vi "WiFi.vi"(0 "New WIFI Name":string="Honor V10", 1 "DelayTime (s)":dbl=1.0 caption="ConfigTime", 3 "配置连接次数":i32=5, 5 "Delay":string="2", 7 "超时时间":u32=25000, 9 "password":string="88888888", 11 "error in":errorcluster caption="error in (no error)", 13 "ping次数":string="6", 14 "ModelNumber":string) -> (4 "Acess":bool, 10 "TotalOut":string, 15 "error out":errorcluster caption="错误输出")   [LabVIEW 2013]
uses:
  <vilib>/Utility/sysdir.llb/System Directory Type.ctl
panel:
  out "数值":i32
  out "Time":u32
  out "新文本":string
  out "原文本":string
  out "STDping":string="WIFI名："
  out "standard output  2":string caption="标准输出"
  out "standard output  3":string caption="标准输出"
  out "SD":path caption="系统目录"
  out "standard output":string caption="标准输出"
  # "第一步，断开相应WIFI的连接\n第二步，替换配置文件\n第三步，添加配置文件到系统\n第四步，连接对应WIFI\n第五步，ping百度网址\n第六步，断开WIFI网络连接"
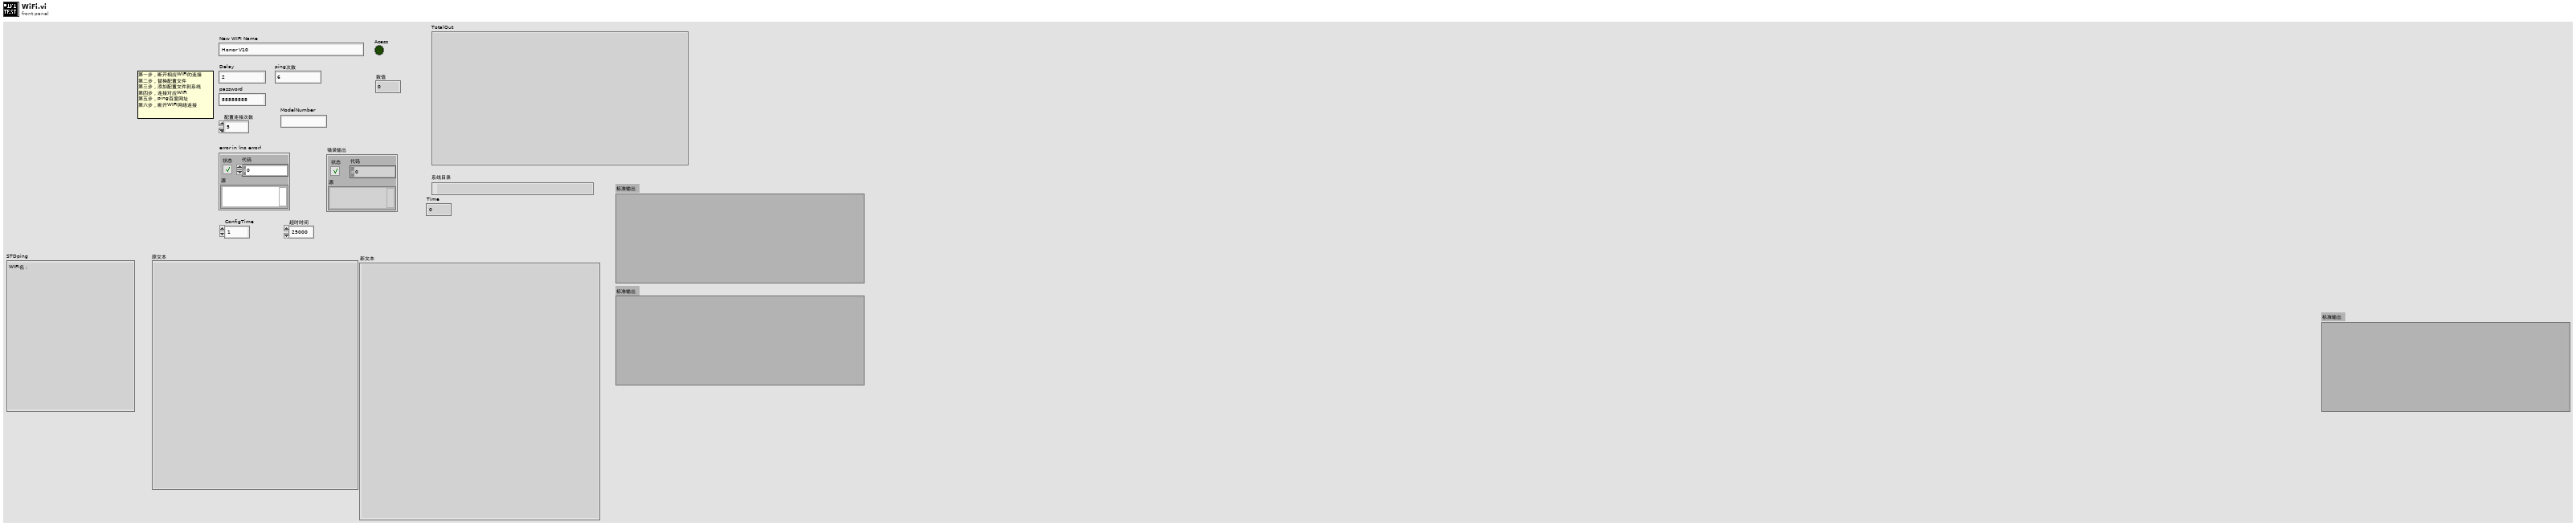
[diagram p1: front panel]
types:
  T1 = typedef "System Directory Type.ctl" = i32
  T2 = enum16{"open", "replace", "create", "open or create", "replace or create", "replace or create with confirmation"}
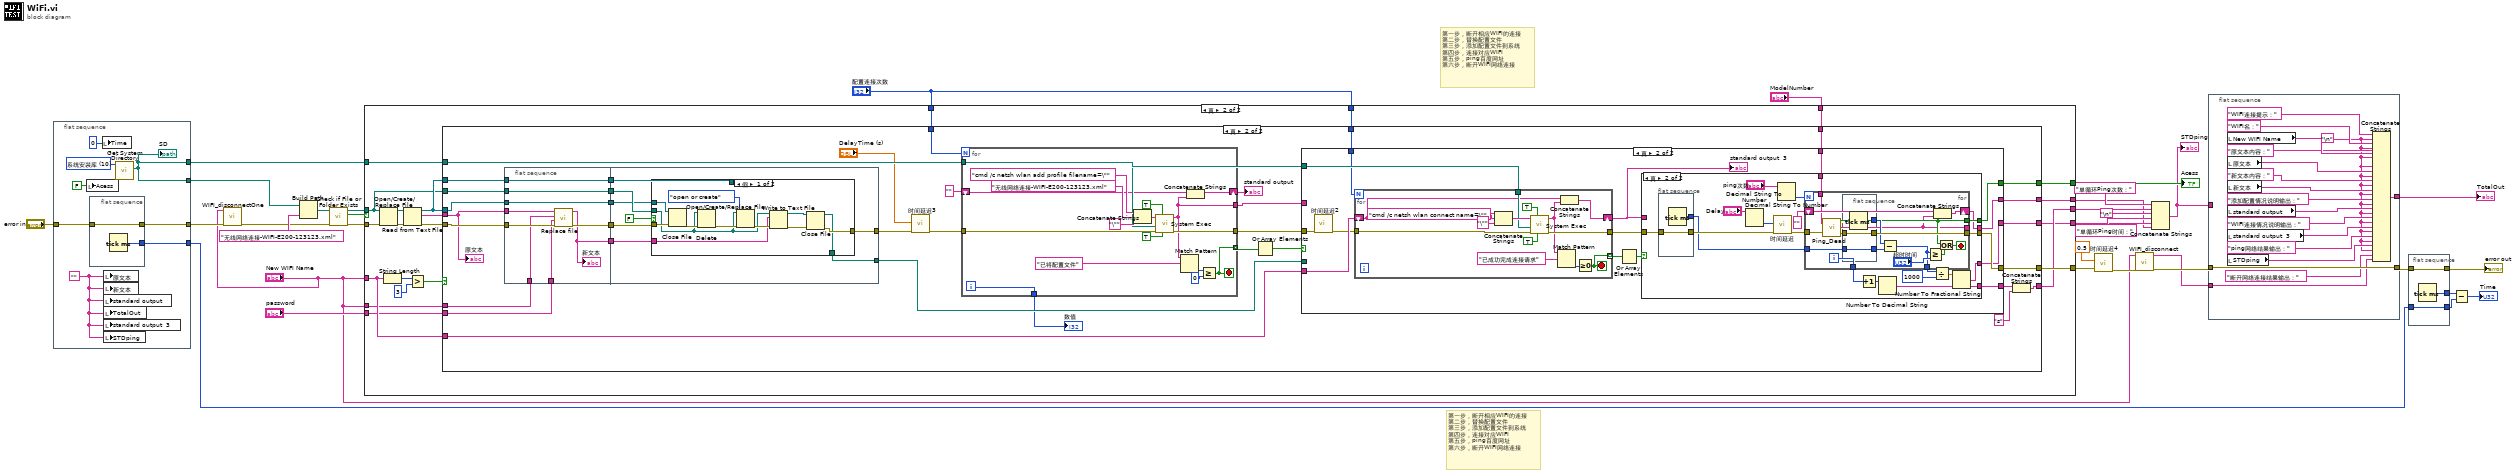
[diagram p0: block diagram]
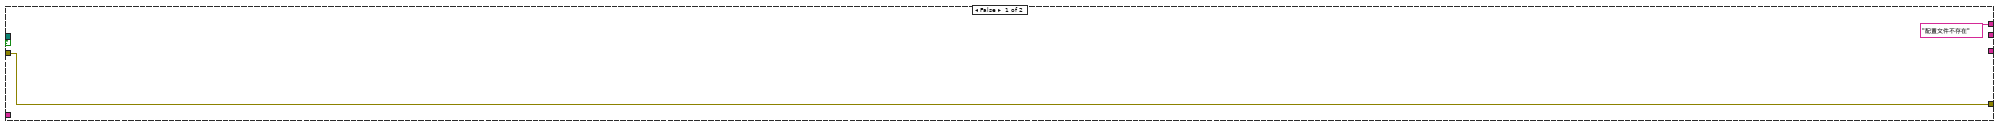
[diagram p2: hidden frame]
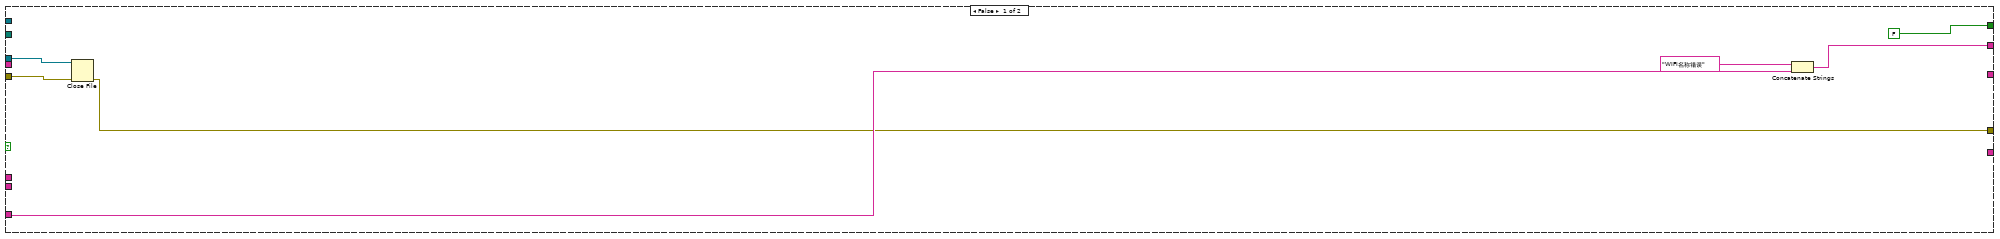
[diagram p3: hidden frame]
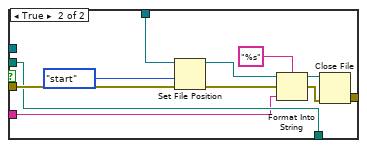
[diagram p4: hidden frame]
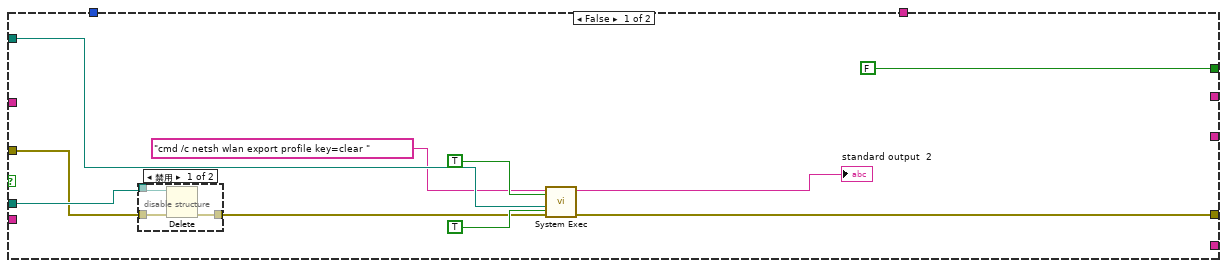
[diagram p5: hidden frame]
diagram:
  # "第一步，断开相应WIFI的连接\n第二步，替换配置文件\n第三步，添加配置文件到系统\n第四步，连接对应WIFI\n第五步，ping百度网址\n第六步，断开WIFI网络连接"
  # "第一步，断开相应WIFI的连接\n第二步，替换配置文件\n第三步，添加配置文件到系统\n第四步，连接对应WIFI\n第五步，ping百度网址\n第六步，断开WIFI网络连接"
  n1 = flat-sequence {
    tunnel: [w41] -> w31
    tunnel: [w41] -> w29
    tunnel: "error in" -> [w38]
    tunnel: [w39] -> w7
    tunnel: [w37] -> w16
    frame #0 {
      w40 = ""
      w42 = T1 10 items=["用户目录"=0, "用户桌面"=1, "用户文档"=2, "用户应用程序数据"=3, "用户设置"=4, "用户临时目录"=5, "公共文档"=6, "公共应用程序数据"=7, "公共设置"=8, "公共缓存"=13, "系统核心库"=9, "系统安装库"=10, "应用程序文件"=11, "启动盘根目录"=12] ("system directory type")
      n2 = local write "Acess"(FALSE ("Acess")) -> ()
      n3 = flat-sequence {
        tunnel: [w44] -> w39
        tunnel: w38 -> [w44]
        tunnel: [w43] -> w37
        frame #0 {
          n4 = Tick Count (ms)() -> (millisecond timer value=w43:u32)
        }
      }
      n5 = local write "Time"(u32 0 ("Time")) -> ()
      n6 = local write "原文本"(w40) -> ()
      n7 = local write "新文本"(w40) -> ()
      n8 = local write "standard output"(w40) -> ()
      n9 = local write "TotalOut"(w40) -> ()
      n10 = local write "standard output  3"(w40) -> ()
      n11 = local write "STDping"(w40) -> ()
      n12 = call <vilib>:"Get System Directory.vi"("system directory type"=w42) -> ("system directory"=w41:path)  [unwired: 10 in]
      "SD" <- w41
    }
  }
  n13 = call "WIFI_disconnectOne.vi"("错误输入"=w7, "WIFI_Name"="New WIFI Name") -> ("error out"=w8:errorcluster)  [unwired: 8 in, 1 out]
  n14 = Build Path(base path=w31, name or relative path="无线网络连接-WIFI-E200-123123.xml" ("名称或相对路径")) -> (appended path=w34:path)
  n15 = call <vilib>:"Check if File or Folder Exists.vi"("error in (no error)"=w8, "path"=w34) -> ("error out"=w32:errorcluster, "file or folder exists?"=w26:bool, "dup path"=w27:path)  [unwired: 7 in]
  n16 = case shown="真" w26 {
    tunnel: w32 -> [w45 w65]
    tunnel: w29 -> [_ w63]
    tunnel: "New WIFI Name" -> [_ w62]
    tunnel: [_ w60] -> w28
    tunnel: ["配置文件不存在" ("standard output") w59] -> w2
    tunnel: [w45 w55] -> w24
    tunnel: w27 -> [_ w54]
    tunnel: "password" -> [_ w53]
    tunnel: "New WIFI Name" -> [_ w52]
    tunnel: "配置连接次数" -> [_ w51]
    tunnel: "配置连接次数" -> [_ w50]
    tunnel: [_ w49] -> w11
    tunnel: [_ w48] -> w3
    tunnel: "ModelNumber" -> [_ w47]
    frame False {
    }
    frame True {
      n17 = Open/Create/Replace File(file path (use dialog)=w54, error in=w65) -> (refnum out=w68:refnum<file>, error out=w67:errorcluster)  [unwired: 4 in, 1 out]
      n18 = String Length(string=w62) -> (length=w58:i32)
      n19 = Read from Text File(file (use dialog)=w68, error in=w67) -> (refnum out=w61:refnum<file>, text=w64:string, error out=w66:errorcluster)  [unwired: 2 in, 1 out]
      n20 = Greater?(x=w58, y=3) -> (0:w56:bool)
      n21 = case shown="真" w56 {
        tunnel: w66 -> [w74 w94]
        tunnel: w61 -> [_ w109]
        tunnel: w64 -> [_ w89]
        tunnel: w62 -> [w73 w107]
        tunnel: w63 -> [_ w106]
        tunnel: w61 -> [w75 w101]
        tunnel: [w69 w105] -> w55
        tunnel: [FALSE ("Acess") w104] -> w60
        tunnel: [w71 w103] -> w59
        tunnel: w54 -> [_ w102]
        tunnel: w53 -> [_ w91]
        tunnel: w52 -> [_ w90]
        tunnel: w51 -> [_ w83]
        tunnel: w50 -> [_ w82]
        tunnel: [_ w78] -> w49
        tunnel: [_ w79] -> w48
        tunnel: w47 -> [_ w76]
        frame False {
          n22 = Close File(refnum=w75, error in=w74) -> (error out=w69:errorcluster)  [unwired: 1 out]
          n23 = Concatenate Strings("WIFI名称错误" ("字符串"), w73) -> (w71:string)
        }
        frame True {
          n24 = flat-sequence {
            tunnel: w101 -> [w134]
            tunnel: w102 -> [w135]
            tunnel: w109 -> [w136]
            tunnel: [w136] -> w97
            tunnel: [w135] -> w96
            tunnel: [w134] -> w95
            tunnel: w94 -> [w133]
            tunnel: [w132] -> w93
            tunnel: [w131] -> w92
            tunnel: w91 -> [w130]
            tunnel: w90 -> [w129]
            tunnel: w89 -> [w128]
            tunnel: [w144] -> w110
            tunnel: [w139] -> w98
            tunnel: w97 -> [w143]
            tunnel: w96 -> [w141]
            tunnel: w95 -> [w140]
            tunnel: w93 -> [w138]
            tunnel: w92 -> [w137]
            frame #0 {
              n25 = call "Replace file.vi"("error in"=w133, "password"=w130, "new wifi name"=w129, "txt input"=w128) -> ("error out"=w132:errorcluster, "txt output"=w131:string)  [unwired: 6 in]
              "新文本" <- w131
            }
            frame #1 {
              n26 = case shown="假" FALSE {
                tunnel: [w148 w162] -> w144
                tunnel: w138 -> [w155 w161]
                tunnel: w143 -> [_ w160]
                tunnel: w141 -> [w147 w158]
                tunnel: w140 -> [w156 _]
                tunnel: [w146 w158] -> w139
                tunnel: w137 -> [w145 w157]
                frame False {
                  n27 = Close File(refnum=w156, error in=w155) -> (error out=w154:errorcluster)  [unwired: 1 out]
                  n28 = Delete(path (use dialog)=w147, error in=w154) -> (error out=w152:errorcluster)  [unwired: 3 in, 2 out]
                  n29 = Open/Create/Replace File(file path (use dialog)=w147, error in=w152, operation (0:open)=T2."open or create" ("操作(0:open)")) -> (error out=w151:errorcluster)  [unwired: 3 in, 2 out]
                  n30 = Write to Text File(file (use dialog)=w147, text=w145, error in=w151) -> (refnum out=w150:refnum<file>, error out=w149:errorcluster)  [unwired: 1 in, 1 out]
                  n31 = Close File(refnum=w150, error in=w149) -> (path=w146:path, error out=w148:errorcluster)
                }
                frame True {
                  n32 = Set File Position(refnum=w160, from (0:start)=enum16{"start", "end", "current"}."start" ("自（0:起始）"), error in=w161) -> (refnum out=w163:refnum<file>, error out=w166:errorcluster)  [unwired: 1 in]
                  n33 = Format Into String(format string="%s" ("格式字符串"), initial string=w163, error in=w166, w157) -> (resulting string=w159:refnum<file>, error out=w165:errorcluster)
                  n34 = Close File(refnum=w159, error in=w165) -> (error out=w162:errorcluster)  [unwired: 1 out]
                }
              }
            }
          }
          n35 = call "时间延迟3"("error in (no error)"=w110, "Delay Time (s)"="DelayTime (s)") -> ("error out"=w100:errorcluster)  [unwired: 9 in]
          n36 = for {
            N: w83 -> [_]
            tunnel: [w121] -> w108
            tunnel: w106 -> [w120]
            tunnel: w100 -> [w119]
            shift-right: [w117] -> w87
            shift-left: "" -> [w118]
            tunnel: [w116] -> w84
            tunnel: [w112] -> w86 mode=indexing
            tunnel: [w111] -> w81
            i -> [w111]
            stop <- w112 stop-if-true
            n37 = Concatenate Strings("cmd /c netsh wlan add profile filename=\"" ("command line"), "无线网络连接-WIFI-E200-123123.xml" ("名称或相对路径"), "\"" ("字符串")) -> (w125:string)
            n38 = call <vilib>:"System Exec.vi"("run minimized? (F)"=TRUE, "wait until completion? (T)"=TRUE, "error in (no error)"=w119, "working directory"=w120, "command line"=w125) -> ("error out"=w121:errorcluster, "standard output"=w116:string)  [unwired: 3 in, 2 out]
            n39 = Match Pattern(string=w116, regular expression="已将配置文件") -> (offset past match=w114:i32)  [unwired: 1 in, 3 out]
            n40 = Concatenate Strings(w118, w116) -> (w117:string)
            n41 = Greater Or Equal?(x=w114, y=0) -> (x >= y?=w112:bool)
          }
          "standard output" <- w87
          "数值" <- w81
          n42 = Or Array Elements(Boolean array=w86) -> (logical OR=w85:bool)
          n43 = case shown="真" w85 {
            tunnel: w108 -> [w169 w189]
            tunnel: [w171 w195] -> w105
            tunnel: [FALSE ("Acess") w194] -> w104
            tunnel: [_ w193] -> w103
            tunnel: w107 -> [_ w191]
            tunnel: w106 -> [w173 w190]
            tunnel: w98 -> [w170 _]
            tunnel: w84 -> [_ _]
            tunnel: w82 -> [_ w187]
            tunnel: [_ w183] -> w80
            tunnel: [_ w182] -> w79
            tunnel: w76 -> [_ w181]
            frame False {
              n44 = disable-structure shown="禁用" {
                disable-tunnel: w170 -> [w180 _]
                disable-tunnel: w169 -> [w179 _]
                disable-tunnel: [w178 _] -> w168
                frame Disabled {
                  n45 = Delete(path (use dialog)=w180, error in=w179) -> (error out=w178:errorcluster)  [unwired: 3 in, 2 out]
                }
                frame Enabled {
                }
              }
              n46 = call <vilib>:"System Exec.vi"("run minimized? (F)"=TRUE, "wait until completion? (T)"=TRUE, "error in (no error)"=w168, "working directory"=w173, "command line"="cmd /c netsh wlan export profile key=clear ") -> ("error out"=w171:errorcluster, "standard output"=→"standard output  2":string)  [unwired: 3 in, 2 out]
            }
            frame True {
              n47 = call "时间延迟2"("error in (no error)"=w189) -> ("error out"=w188:errorcluster)  [unwired: 10 in]
              n48 = for {
                N: w187 -> [_]
                tunnel: [w249] -> w192
                tunnel: w190 -> [w245]
                tunnel: w188 -> [w244]
                shift-right: [w243] -> w186
                shift-left: w191 -> [w242]
                tunnel: [w238] -> w185 mode=indexing
                stop <- w238 stop-if-true
                n49 = Concatenate Strings("cmd /c netsh wlan connect name=\"" ("command line"), w242, "\"" ("字符串")) -> (w246:string)
                n50 = call <vilib>:"System Exec.vi"("run minimized? (F)"=TRUE, "wait until completion? (T)"=TRUE, "error in (no error)"=w244, "working directory"=w245, "command line"=w246) -> ("error out"=w249:errorcluster, "standard output"=w241:string)  [unwired: 3 in, 2 out]
                n51 = Match Pattern(string=w241, regular expression="已成功完成连接请求") -> (offset past match=w239:i32)  [unwired: 1 in, 3 out]
                n52 = Concatenate Strings(w242, w241) -> (w243:string)
                n53 = Greater Or Equal To 0?(x=w239) -> (x >= 0?=w238:bool)
              }
              "standard output  3" <- w186
              n54 = Or Array Elements(Boolean array=w185) -> (logical OR=w184:bool)
              n55 = case shown="真" w184 {
                tunnel: [w196 w215] -> w195
                tunnel: [_ w214] -> w194
                tunnel: [_ w205] -> w193
                tunnel: w192 -> [w196 w208]
                tunnel: w186 -> [_ _]
                tunnel: [_ w203] -> w183
                tunnel: [_ w198] -> w182
                tunnel: w181 -> [_ w197]
                frame False {
                }
                frame True {
                  n56 = flat-sequence {
                    tunnel: [w218] -> w209
                    tunnel: w208 -> [w218]
                    tunnel: [w217] -> w207
                    frame #0 {
                      n57 = Tick Count (ms)() -> (millisecond timer value=w217:u32)
                    }
                  }
                  n58 = Decimal String To Number(string="Delay") -> (number=w213:i32)  [unwired: 2 in, 1 out]
                  n59 = call "时间延迟"("error in (no error)"=w209, "Delay Time (s)"=w213) -> ("error out"=w216:errorcluster)  [unwired: 9 in]
                  n60 = Decimal String To Number(string="ping次数") -> (number=w210:i32)  [unwired: 2 in, 1 out]
                  n61 = for {
                    N: w210 -> [_]
                    tunnel: w216 -> [w234]
                    tunnel: [w232] -> w215
                    tunnel: [w226] -> w214
                    tunnel: [w223] -> _
                    tunnel: w207 -> [w229]
                    shift-right: [w222] -> w205
                    shift-left: "" -> [w224]
                    tunnel: [w221] -> w204
                    tunnel: [w220] -> w201
                    tunnel: w197 -> [w219]
                    i -> [w221]
                    stop <- w227 stop-if-true
                    n62 = call "Ping_Dead.vi"("ModelNumber"=w219, "error in"=w234) -> ("Acess"=w226:bool, "standard output"=w223:string, "error out"=w233:errorcluster)
                    n63 = flat-sequence {
                      tunnel: w233 -> [w237]
                      tunnel: [w237] -> w232
                      tunnel: [w236] -> w231
                      tunnel: [w235] -> w230
                      tunnel: w229 -> [w235]
                      frame #0 {
                        n64 = Tick Count (ms)() -> (millisecond timer value=w236:u32)
                      }
                    }
                    n65 = Subtract(x=w231, y=w230) -> (x-y=w220:u32)
                    n66 = Greater Or Equal?(x=w220, y="超时时间") -> (x >= y?=w225:bool)
                    n67 = Concatenate Strings(w224, w223) -> (w222:string)
                    n68 = Or(x=w226, y=w225) -> (x .or. y?=w227:bool)
                  }
                  n69 = Increment(x=w204) -> (x+1=w202:i32)
                  n70 = Number To Decimal String(number=w202) -> (decimal integer string=w203:string)  [unwired: 1 in]
                  n71 = Divide(x=w201, y=u32 1000) -> (x/y=w199:dbl)
                  n72 = Number To Fractional String(number=w199) -> (F-format string=w198:string)  [unwired: 3 in]
                }
              }
            }
          }
          n73 = Concatenate Strings(w80, "s") -> (w78:string)
          "原文本" <- w89
        }
      }
    }
  }
  "Acess" <- w28
  n74 = call "时间延迟4"("error in (no error)"=w24, "Delay Time (s)"=0.5) -> ("error out"=w23:errorcluster)  [unwired: 9 in]
  n75 = call "WIFI_disconnect.vi"("错误输入"=w23, "WIFI_Name"="New WIFI Name") -> ("error out"=w19:errorcluster, "standard output  2"=w5:string)  [unwired: 8 in]
  n76 = Concatenate Strings("单循环Ping次数：", w11, "\n", "单循环Ping时间：", w3, w2) -> (w12:string)
  "STDping" <- w12
  n77 = flat-sequence {
    tunnel: w12 -> [_]
    tunnel: [w255] -> w25
    tunnel: w19 -> [w254]
    tunnel: [w254] -> w17
    tunnel: w5 -> [w252]
    frame #0 {
      w256 = "\n"
      n78 = local read "New WIFI Name"() -> (w267:string)
      n79 = local read "原文本"() -> (w265:string)
      n80 = local read "新文本"() -> (w263:string)
      n81 = local read "standard output"() -> (w261:string)
      n82 = local read "standard output  3"() -> (w259:string)
      n83 = local read "STDping"() -> (w257:string)
      n84 = Concatenate Strings("WIFI连接提示：", w256, "WIFI名：", w256, w267, w256, "原文本内容：", w256, w265, w256, "新文本内容：", w256, w263, w256, "添加配置情况说明输出：", w256, w261, w256, "WIFI连接情况说明输出：", w256, w259, w256, "ping网络结果输出：", w256, w257, w256, "断开网络连接结果输出：", w252) -> (w255:string)
    }
  }
  n85 = flat-sequence {
    tunnel: [w272] -> w18
    tunnel: w17 -> [w272]
    tunnel: w16 -> [w270]
    tunnel: [w271] -> w15
    tunnel: [w270] -> w14
    frame #0 {
      n86 = Tick Count (ms)() -> (millisecond timer value=w271:u32)
    }
  }
  n87 = Subtract(x=w15, y=w14) -> (x-y=→"Time":u32)
  "TotalOut" <- w25
  "error out" <- w18
